vi "test_fpga_sid_v2.vi"() -> ()   [LabVIEW 2016]
uses:
  <vilib>/Platform/TimedLoop/XDataNode/timing_clust.ctl
  <vilib>/Platform/TimedLoop/XDataNode/nitl_modes.ctl
  <vilib>/Platform/TimedLoop/XDataNode/wakeup.ctl
  <vilib>/rvi/Emulation/niFpgaSctlEmulationGetInTimedLoop.vi
  <vilib>/rvi/Emulation/niFpgaEmulationReportErrorSimple.vi
  <vilib>/rvi/Emulation/niFpgaGetClockAttributes.vi
  <vilib>/rvi/Emulation/niFpgaCriticalErrorInLSC.vi
  <vilib>/rvi/Emulation/niFpgaProcessEmulError.vi
  <vilib>/rvi/Memory/Memory_Emulation/nirvimemoryFastEmulation.vi
  <vilib>/rvi/Memory/Memory_Emulation/nirvimemoryEmulation.vi
  <vilib>/rvi/Emulation/niFpgaEmulationIsFPGAContextNoSignature.vi
  <vilib>/rvi/DataTransferAndStorage/Container/Common/niFpgaContainerGetUniqueNameForEmu.vi
  <vilib>/rvi/errors/nirviReportUnexpectedCaseInternalError (U32).vi
  <vilib>/Platform/TimedLoop/XDataNode/XDataNode.xnode
  <vilib>/rvi/DataTransferAndStorage/Container/XNode/niFpgaContainer.xnode
  <vilib>/Platform/TimedLoop/XDataNode/XDNodeRunTimeDep.lvlib
panel:
  in  "sid.p.params":T1={"sysIdOutputRate"=100, "sysIdWaveSize"=4092, "sysIdRepetitions"=50} {"sysIdOutputRate" min=10}
  out "sid.o.count":u16
  out "sid.s.running":bool
  in  "sid.p.start":bool
  in  "sid.i.height":fxp<+/-,31,4>
  in  "inputValid":bool
  out "outputValid":bool
  in  "sid.m.motion":cluster{"write":bool, "data":i16, "index":u16}
  out "sid.o.height":fxp<+/-,43,16>
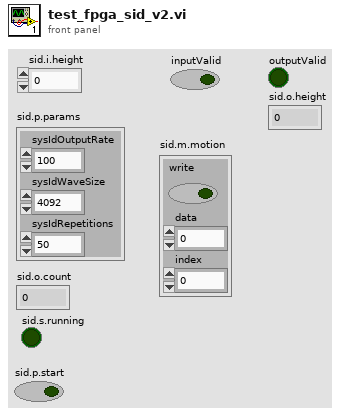
[diagram p1: front panel]
types:
  T1 = cluster{"sysIdOutputRate":u16, "sysIdWaveSize":u16, "sysIdRepetitions":u16}
  T2 = typedef "XDNodeRunTimeDep.lvlib/timing_clust.ctl" = cluster{"Expected End [f-1]":u64, "Actual End [f-1]":u64, "Finished Late? [f-1]":bool, "Expected End [i-1]":u64, "Actual End [i-1]":u64, "Finished Late? [i-1]":bool, "Expected Start [i]":u64, "Actual Start [i]":u64, "Expected Start [f]":u64, "Actual Start [f]":u64, "Source Name":string, "Structure Name":string, "Period":i64, "Deadline":i64, "Offset":i64, "Start":i64, "Priority":i32, "Timeout":i32, "Mode":T3, "Wakeup Reason":T4, "Error":errorcluster, "Source Type":string, "Secondary Source Type":string, "Global End Time":u64, "Global Start Time":u64, "Frame Duration":u64, "Iteration Duration":u64, "Assigned CPU":i32, "I/O Scan Engine Mode":u32}
  T3 = typedef "XDNodeRunTimeDep.lvlib/nitl_modes.ctl" = enum32{"No Change", "Process missed periods, maintain original phase", "Discard missed periods, maintain original phase", "Process missed periods, ignore original phase", "Discard missed periods, ignore original phase"}
  T4 = typedef "XDNodeRunTimeDep.lvlib/wakeup.ctl" = enum32{"Normal", "Aborted", "Asynchronous wakeup", "Timing source error", "Timed loop error", "Timeout"}
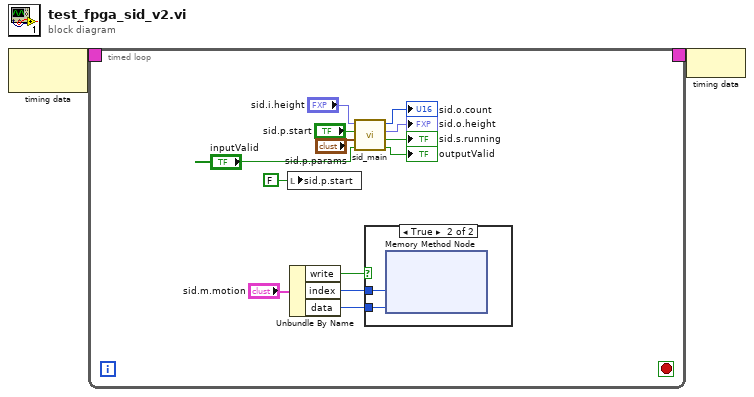
[diagram p0: block diagram]
diagram:
  n1 = node-c288() -> (w2:T2)  [unwired: 1 in]
  n2 = timed-loop {
    timing: w2 -> [_]
    timing-out: [_] -> w1
    stop <- _ stop-if-true
    n3 = local write "sid.p.start"(FALSE ("sid.p.start")) -> ()
    n4 = Unbundle By Name("sid.m.motion") -> ("write"=w5:bool, "index"=w6:u16, "data"=w7:i16)
    n5 = call "sid_main.vi"("inputValid"="inputValid", "sid.p.params"="sid.p.params", "sid.p.start"="sid.p.start", "sid.i.height"="sid.i.height") -> ("outputValid"=→"outputValid":bool, "sid.running"=→"sid.s.running":bool, "sid.o.height"=→"sid.o.height":fxp<+/-,43,16>, "sid.o.count"=→"sid.o.count":u16)  [unwired: 4 in]
    n6 = case shown="True" w5 {
      tunnel: w6 -> [_ w17]
      tunnel: w7 -> [_ w16]
      frame False {
      }
      frame True {
        n7 = xnode ("Memory Method Node")("Address"=w17, "Data"=w16) -> ()  [unwired: 1 in, 1 out]
      }
    }
  }
  n8 = node-c288(w1) -> ()
